vi "GetIONameReference.vi"(8 "error in":errorcluster, 11 "IOName in":refnum<class "IOName.lvclass">) -> (0 "error out":errorcluster, 1 "IOName reference":refnum<vi>, 3 "IOName out":refnum<class "IOName.lvclass">)   [LabVIEW 2014, in "IOName.lvclass"]
uses:
  IOName.lvclass
  Generic/Generic.lvclass
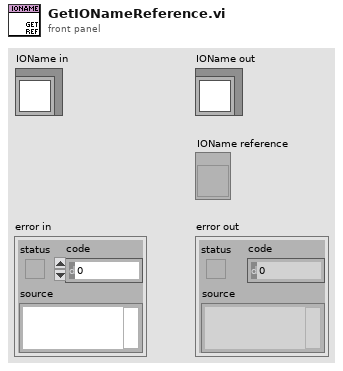
[diagram p1: front panel]
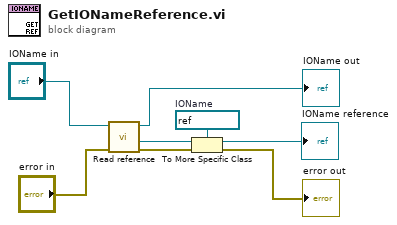
[diagram p0: block diagram]
diagram:
  w4 = refnum<vi> refnum  # IOName
  n1 = call "Read reference.vi"("error in"="error in", "GObject in"="IOName in") -> ("error out"=w5:errorcluster, "reference"=w6:refnum<vi>, "GObject out"=→"IOName out":refnum<class "IOName.lvclass">)  [unwired: 5 in]
  n2 = To More Specific Class(target class=w4, reference=w6, error in=w5) -> (specific class reference=→"IOName reference":refnum<vi>, error out=→"error out":errorcluster)
